vi "9_Check no is Even or Odd.vi"() -> ()   [LabVIEW 2018]
panel:
  out "Boolean 2":bool
  out "Boolean":bool
  in  "INPUT NUMBER":dbl
  # "WAP to find a given number is EVEN or ODD"
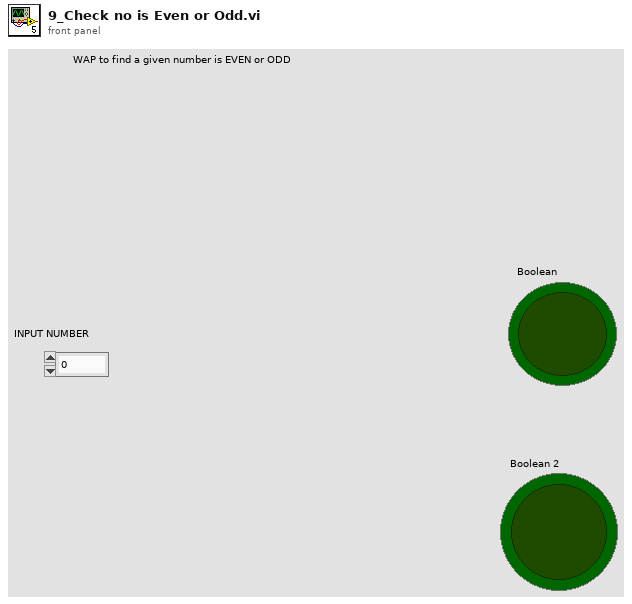
[diagram p1: front panel]
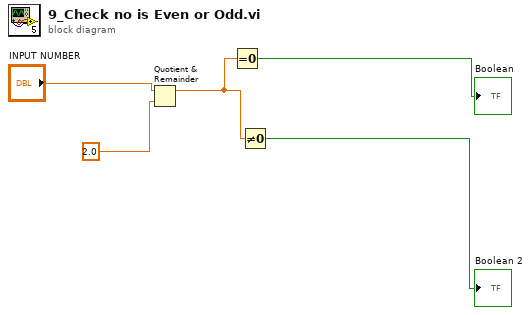
[diagram p0: block diagram]
diagram:
  n1 = Quotient & Remainder(x="INPUT NUMBER", y=2.0 ("floor(x/y)")) -> (x-y*floor(x/y)=w3:dbl)  [unwired: 1 out]
  n2 = Equal To 0?(x=w3) -> (x = 0?=→"Boolean":bool)
  n3 = Not Equal To 0?(x=w3) -> (x != 0?=→"Boolean 2":bool)
